vi "Main.vi"() -> ()   [LabVIEW 2020]
uses:
  <vilib>/Instr/_visa.llb/VISA Find Search Mode.ctl
  <vilib>/Platform/TimedLoop/XDataNode/timing_clust.ctl
  <vilib>/Platform/TimedLoop/XDataNode/nitl_modes.ctl
  <vilib>/Platform/TimedLoop/XDataNode/wakeup.ctl
  <vilib>/Platform/TimedLoop/scheduler/LVUserAPI/_suppVIs/Create_SoftwareTrigger_TSource.vi
  <vilib>/Platform/TimedLoop/scheduler/LVUserAPI/_suppVIs/Create_1kHz_TSource.vi
  <vilib>/platform/TimedLoop/XDataNode/XDataNode.xnode
  <vilib>/Platform/TimedLoop/XDataNode/XDNodeRunTimeDep.lvlib
panel:
  in  "Relay Mode":bool
  out "v1_1 13":bool=TRUE
  out "v1_1 12":bool=TRUE
  out "v1_1 11":bool=TRUE
  out "v1_1 10":bool=TRUE
  out "v1_1 9":bool=TRUE
  out "v1_1 8":bool=TRUE
  out "v1_1 7":bool=TRUE
  out "v1_1 6":bool=TRUE
  out "v1_1 5":bool=TRUE
  out "v1_1 4":bool=TRUE
  out "v1_1 3":bool=TRUE
  out "v1_1 2":bool=TRUE
  out "N2 4":bool caption="N2 2"
  out "N2 5":bool caption="N2 2"
  out "N2 3":bool caption="N2 2"
  out "Gas 11":bool
  out "Gas 10":bool
  out "Gas 9":bool
  out "H2O":bool
  out "CO2":bool
  out "CO":bool
  out "С2Н6":bool
  out "С2Н4":bool
  out "С2Н2":bool
  out "CH4":bool
  out "N2":bool
  out "v12_11":bool
  out "v12_10":bool
  out "v12_9":bool
  out "v12_8":bool
  out "v12_7":bool
  out "v12_6":bool
  out "v12_5":bool
  out "v12_4":bool
  out "v12_3":bool
  out "v12_2":bool
  out "v12_1":bool
  out "v4":bool
  out "flow 2":dbl format="%#.1f"
  out "v3_1":bool
  out "v3_2":bool
  out "v3_3":bool
  out "v2_3":bool
  out "v2_2":bool
  out "flow 1":dbl format="%#.1f"
  out "v2_1":bool
  out "v1_11":bool
  out "v1_10":bool
  out "v1_9":bool
  out "v1_8":bool
  out "v1_7":bool
  out "v1_6":bool
  out "v1_5":bool
  out "v1_4":bool
  out "v1_3":bool
  out "v1_2":bool
  out "v1_1":bool
  in  "coef":dbl(ring)=0.71 caption="Gas type" items=["NO2"=0.71, "SF6"=0.26]
  in  "Vlv_1 13":bool
  in  "Vlv_1 12":bool
  in  "Vlv_1 9":bool
  in  "Vlv_1 14":bool
  in  "DisableReadback":bool caption="Checkbox"
  out "Time left":i32
  in  "Stop":bool
  in  "Set point":i32
  in  "Play":bool
  in  "flow 2 s":dbl min=0.0 max=1000.0
  in  "flow 1 s":dbl min=0.0 max=500.0
  in  "Apply All":bool
  in  "Connect":bool
  in  "Vlv_1 11":bool
  in  "Vlv_1 8":bool
  in  "Vlv_1 7":bool
  in  "Vlv_1 6":bool
  in  "Vlv_1 5":bool
  in  "Vlv_1 4":bool
  in  "Vlv_1 3":bool
  in  "Vlv_1 2":bool
  in  "Vlv_1":bool
  in  "Vlv_1 10":bool
  out "Status":bool
  in  "CH2_SP":u16 max=999 step=1
  in  "CH1_SP":dbl max=999.0 step=1.0
  out "CH2_FB":u16=1 min=1 max=255 step=1
  out "CH1_FB":dbl=1.0 min=1.0 max=255.0 step=1.0 format="%.1g"
  out "Connection":bool
  out "find list":string[](array[string])
  in  "Port":u16(ring) items=["COM1 - Последовательный порт"]
  # "Current value"
  # "Gas 1 proportion"
  # "Gas 2 proportion"
  # "Current value"
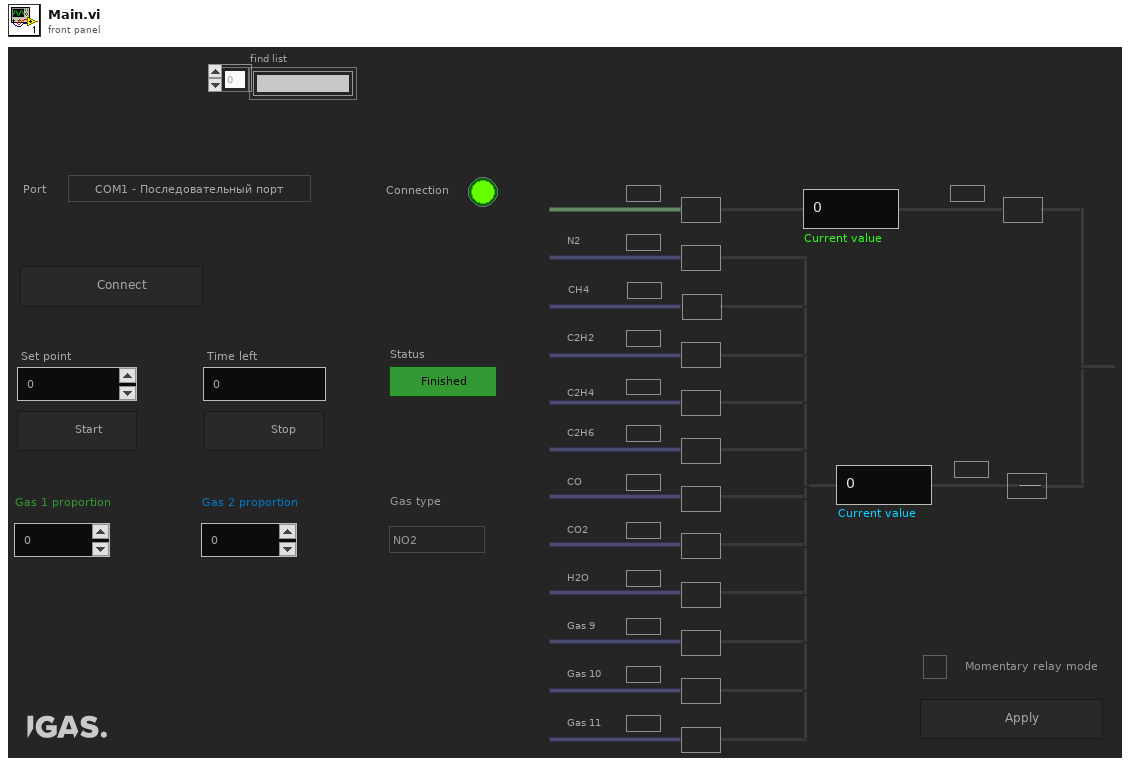
[diagram p1: front panel]
types:
  T1 = typedef "XDNodeRunTimeDep.lvlib/timing_clust.ctl" = cluster{"Expected End [f-1]":u64, "Actual End [f-1]":u64, "Finished Late? [f-1]":bool, "Expected End [i-1]":u64, "Actual End [i-1]":u64, "Finished Late? [i-1]":bool, "Expected Start [i]":u64, "Actual Start [i]":u64, "Expected Start [f]":u64, "Actual Start [f]":u64, "Source Name":string, "Structure Name":string, "Period":i64, "Deadline":i64, "Offset":i64, "Start":i64, "Priority":i32, "Timeout":i32, "Mode":T2, "Wakeup Reason":T3, "Error":errorcluster, "Source Type":string, "Secondary Source Type":string, "Global End Time":u64, "Global Start Time":u64, "Frame Duration":u64, "Iteration Duration":u64, "Assigned CPU":i32, "I/O Scan Engine Mode":u32}
  T2 = typedef "XDNodeRunTimeDep.lvlib/nitl_modes.ctl" = enum32{"No Change", "Process missed periods, maintain original phase", "Discard missed periods, maintain original phase", "Process missed periods, ignore original phase", "Discard missed periods, ignore original phase"}
  T3 = typedef "XDNodeRunTimeDep.lvlib/wakeup.ctl" = enum32{"Normal", "Aborted", "Asynchronous wakeup", "Timing source error", "Timed loop error", "Timeout"}
  T4 = cluster{"Mode":enum16{"RTU", "ASCII"}, "адрес датчика":u16}
  T5 = cluster{"Mode":enum16{"RTU", "ASCII"}, "Slave Address":u8}
  T6 = typedef "VISA Find Search Mode.ctl" = u32
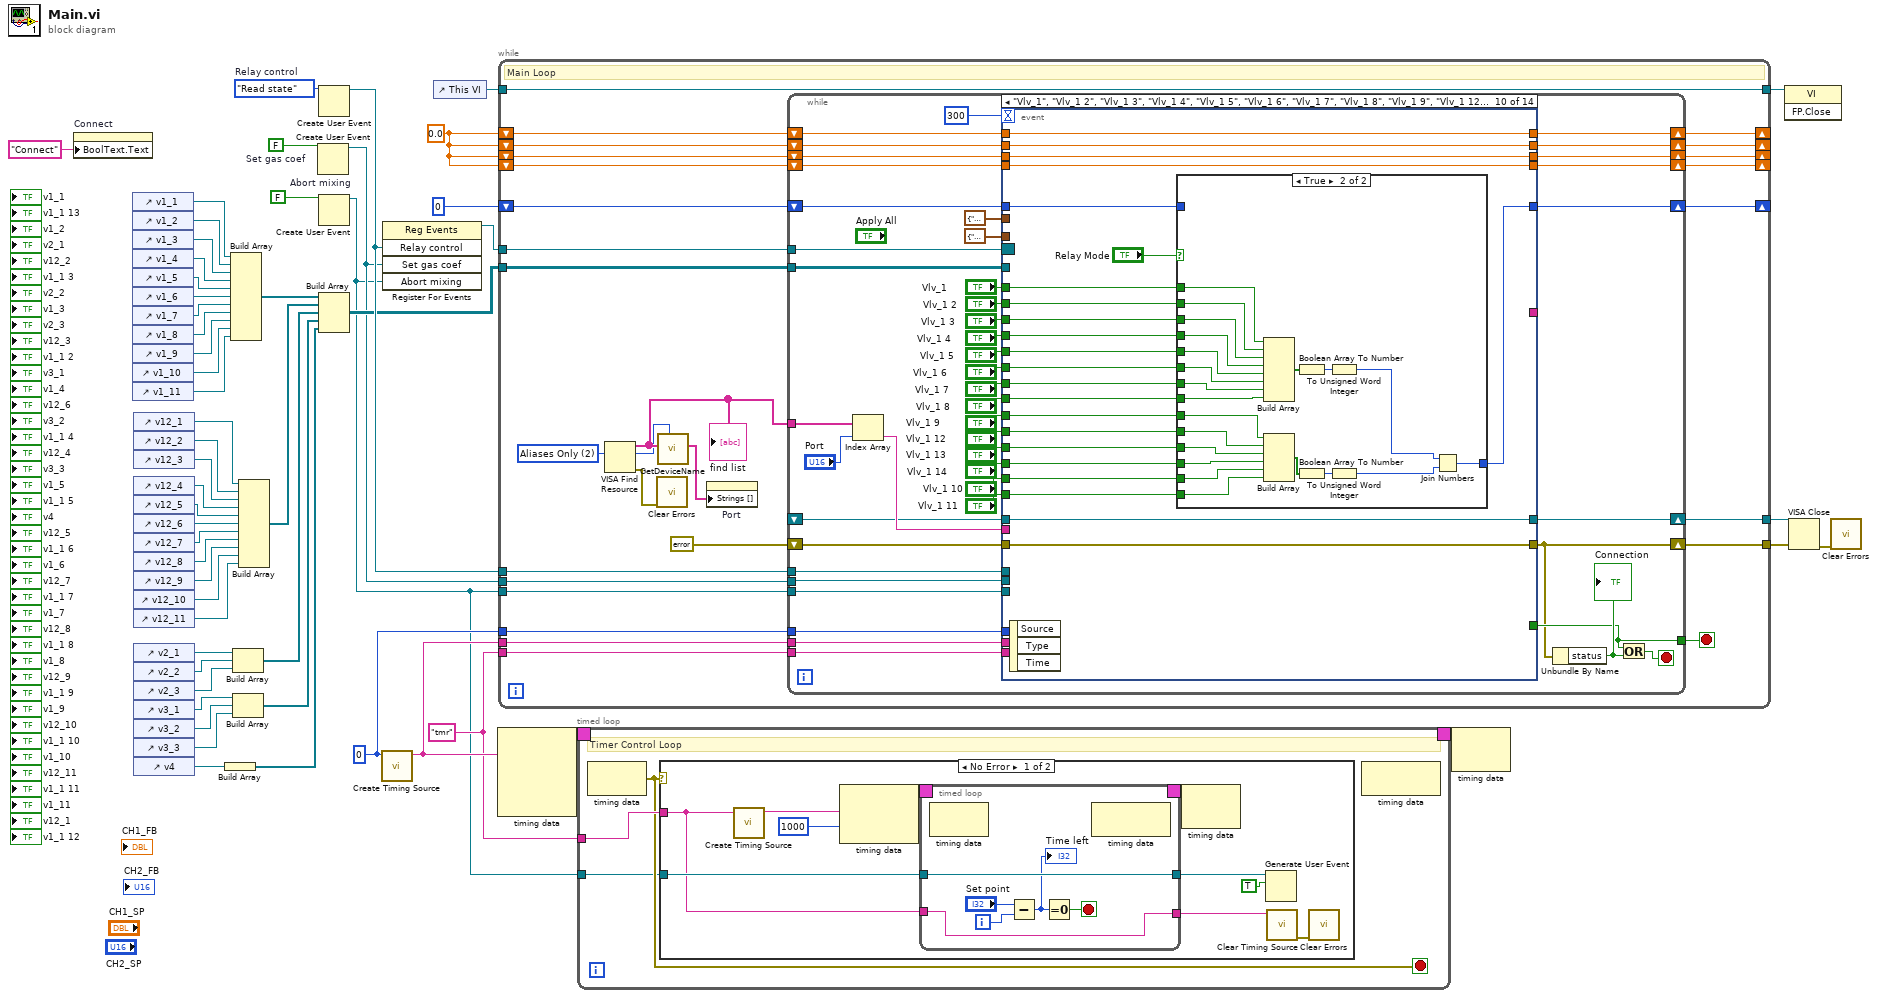
[diagram p0: block diagram]
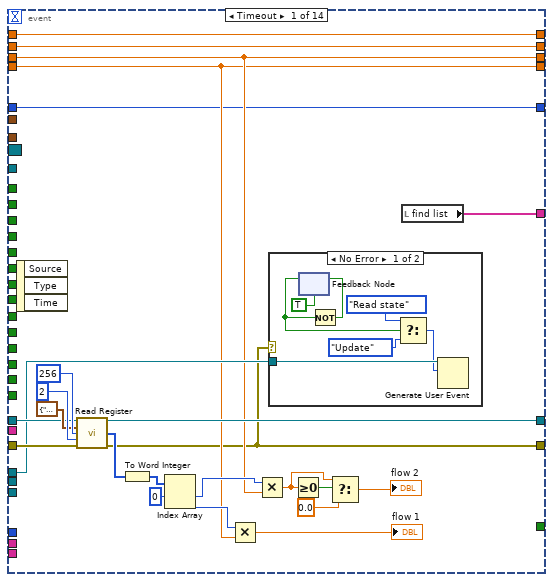
[diagram p3: hidden frame]
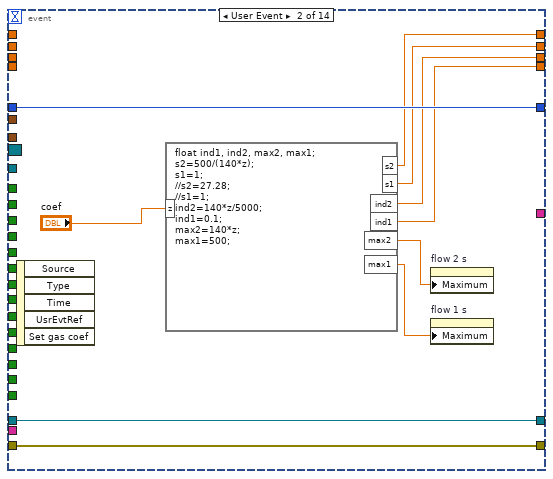
[diagram p5: hidden frame]
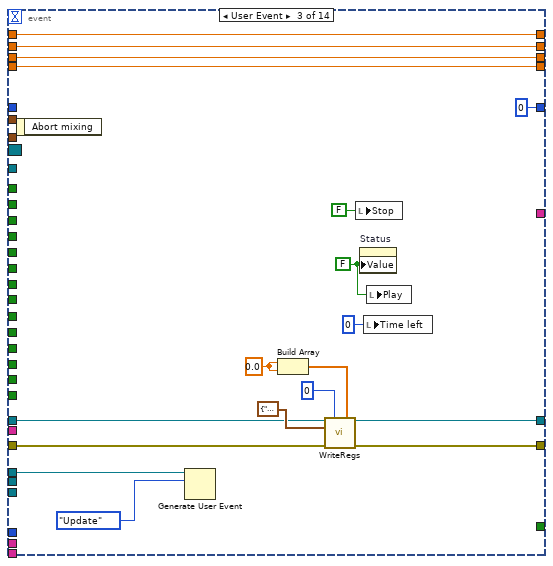
[diagram p6: hidden frame]
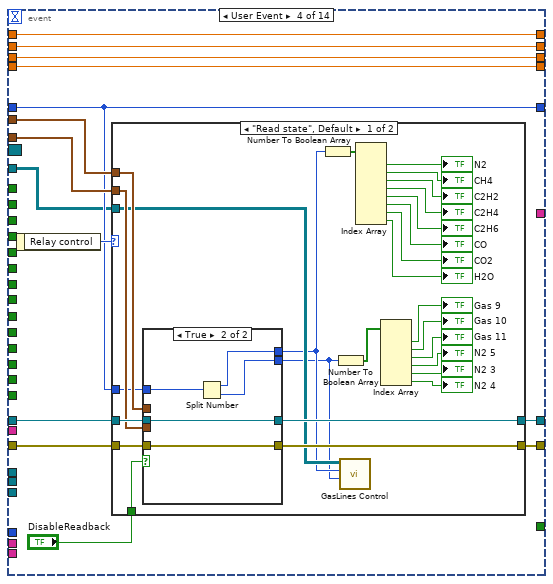
[diagram p7: hidden frame]
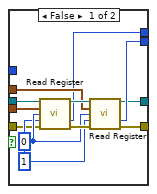
[diagram p8: hidden frame]
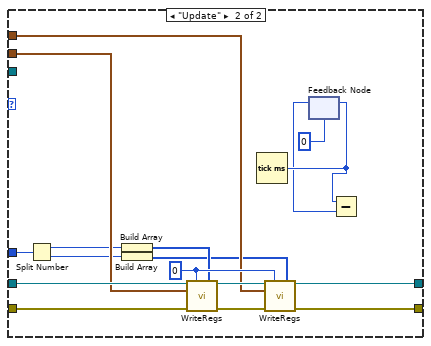
[diagram p9: hidden frame]
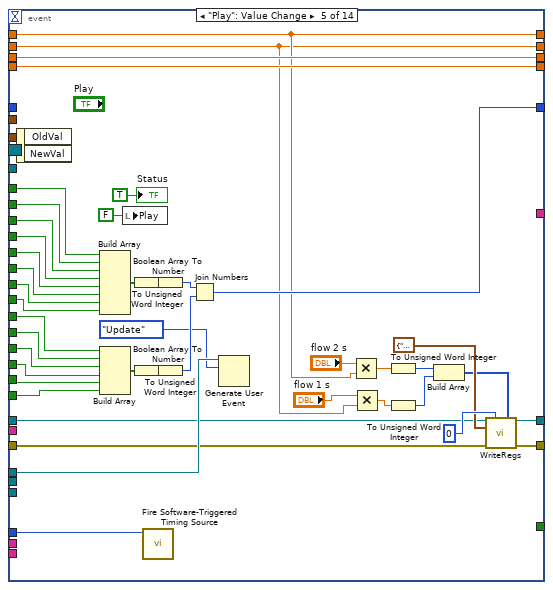
[diagram p10: hidden frame]
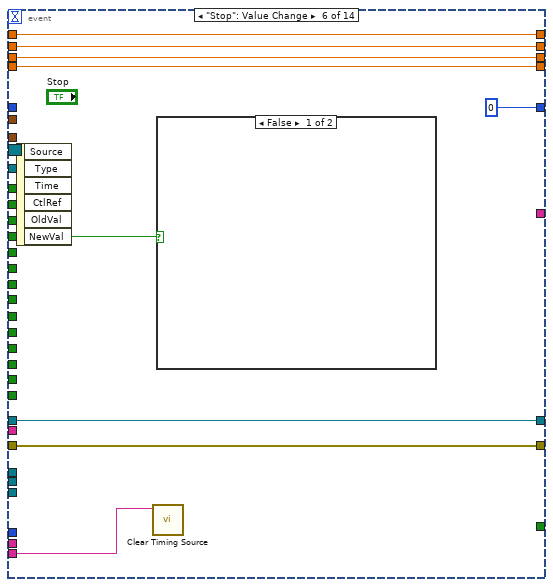
[diagram p11: hidden frame]
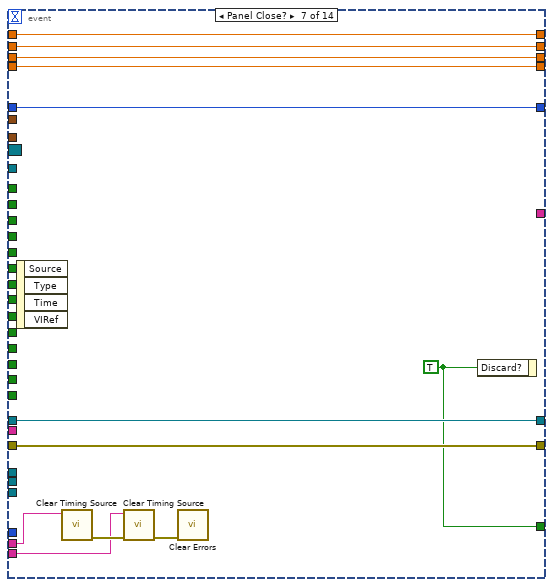
[diagram p13: hidden frame]
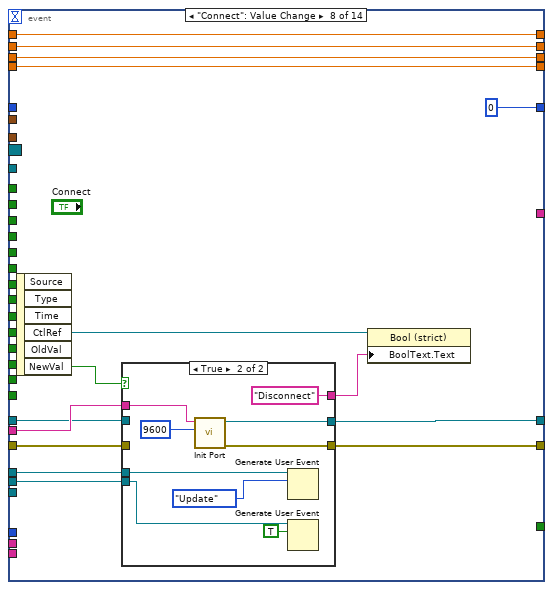
[diagram p14: hidden frame]
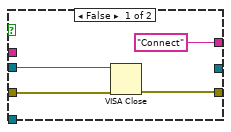
[diagram p15: hidden frame]
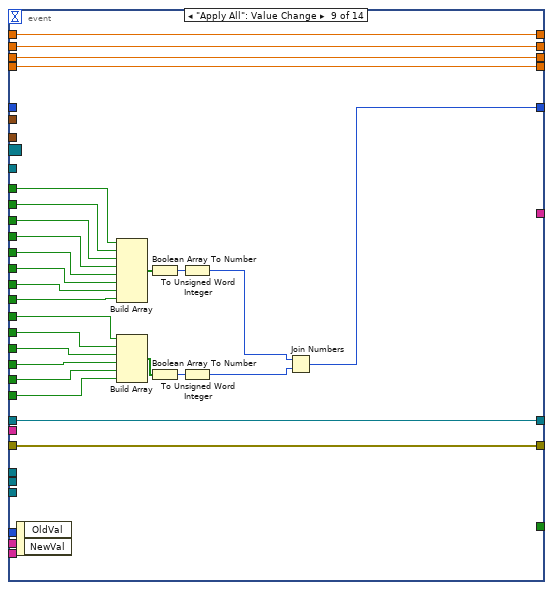
[diagram p16: hidden frame]
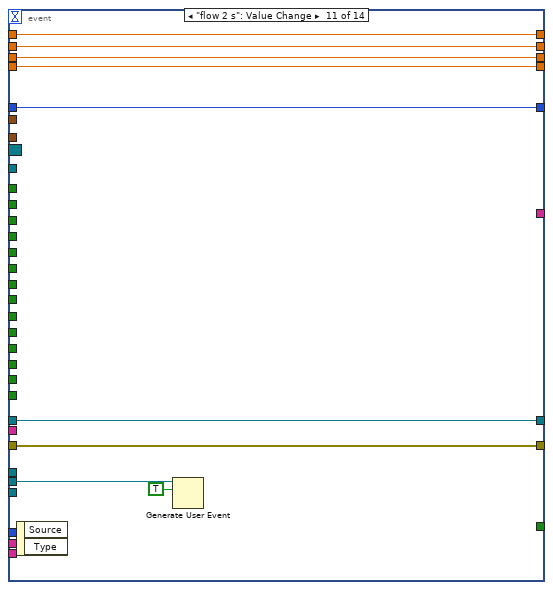
[diagram p18: hidden frame]
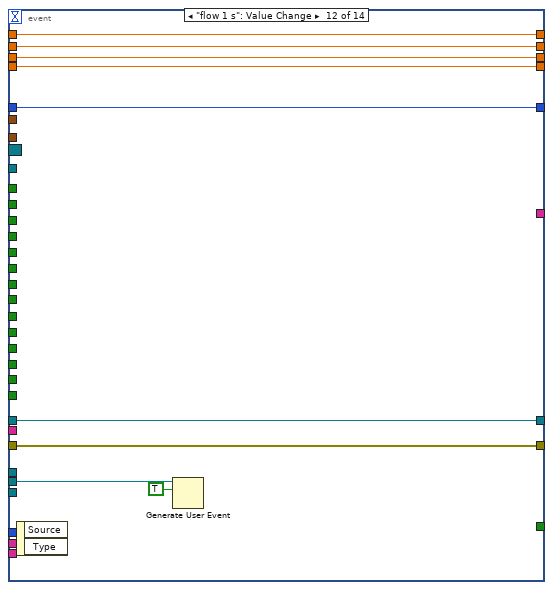
[diagram p19: hidden frame]
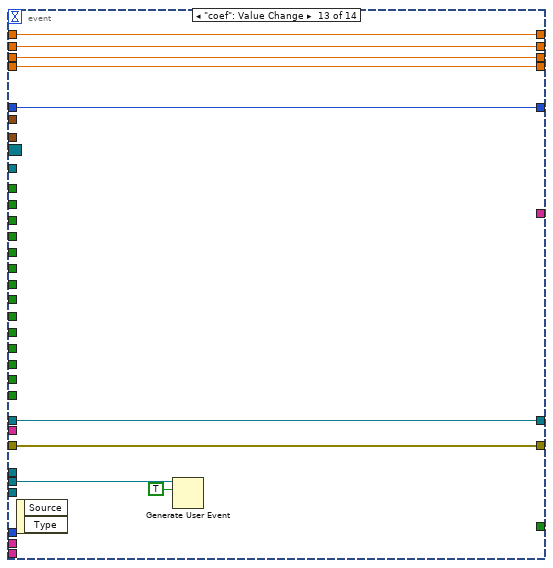
[diagram p20: hidden frame]
diagram:
  w3 = FALSE  # Abort mixing
  w4 = "tmr" ("name (in)")
  w6 = u8 0 ("trigger ID")
  w9 = 0.0 ("s2")
  w10 = FALSE  # Set gas coef
  w51 = enum16{"Read state", "Update"}."Read state"  # Relay control
  n1 = property on="Connect" class="Bool (strict)"("BoolText.Text"="Connect" ("Boolean Text.Text")) -> ()  [unwired: 2 in, 2 out]
  n2 = control-ref of="v1_1"() -> (w41:refnum<vi>)
  n3 = control-ref of="v1_2"() -> (w42:refnum<vi>)
  n4 = control-ref of="v1_3"() -> (w43:refnum<vi>)
  n5 = control-ref of="v1_4"() -> (w44:refnum<vi>)
  n6 = control-ref of="v1_5"() -> (w45:refnum<vi>)
  n7 = control-ref of="v1_6"() -> (w46:refnum<vi>)
  n8 = control-ref of="v1_7"() -> (w40:refnum<vi>)
  n9 = control-ref of="v1_8"() -> (w39:refnum<vi>)
  n10 = control-ref of="v1_9"() -> (w38:refnum<vi>)
  n11 = control-ref of="v1_10"() -> (w37:refnum<vi>)
  n12 = control-ref of="v1_11"() -> (w36:refnum<vi>)
  n13 = control-ref of="v12_1"() -> (w30:refnum<vi>)
  n14 = control-ref of="v12_2"() -> (w31:refnum<vi>)
  n15 = control-ref of="v12_3"() -> (w32:refnum<vi>)
  n16 = control-ref of="v12_4"() -> (w33:refnum<vi>)
  n17 = control-ref of="v12_5"() -> (w34:refnum<vi>)
  n18 = control-ref of="v12_6"() -> (w35:refnum<vi>)
  n19 = control-ref of="v12_7"() -> (w29:refnum<vi>)
  n20 = control-ref of="v12_8"() -> (w28:refnum<vi>)
  n21 = control-ref of="v12_9"() -> (w27:refnum<vi>)
  n22 = control-ref of="v12_10"() -> (w26:refnum<vi>)
  n23 = control-ref of="v12_11"() -> (w25:refnum<vi>)
  n24 = control-ref of="v2_1"() -> (w21:refnum<vi>)
  n25 = control-ref of="v2_2"() -> (w20:refnum<vi>)
  n26 = control-ref of="v2_3"() -> (w19:refnum<vi>)
  n27 = control-ref of="v3_1"() -> (w18:refnum<vi>)
  n28 = control-ref of="v3_2"() -> (w17:refnum<vi>)
  n29 = control-ref of="v3_3"() -> (w16:refnum<vi>)
  n30 = control-ref of="v4"() -> (w15:refnum<vi>)
  n31 = Build Array(w15) -> (w12:refnum<vi>[])
  n32 = Build Array(w41, w42, w43, w44, w45, w46, w40, w39, w38, w37, w36) -> (w24:refnum<vi>[])
  n33 = Build Array(w21, w20, w19) -> (w14:refnum<vi>[])
  n34 = Build Array(w18, w17, w16) -> (w13:refnum<vi>[])
  n35 = Build Array(w30, w31, w32, w33, w34, w35, w29, w28, w27, w26, w25) -> (w23:refnum<vi>[])
  n36 = Create User Event(user event datatype=w10) -> (user event=w2:refnum<user-event>)  [unwired: 1 in, 1 out]
  n37 = Create User Event(user event datatype=w51) -> (user event=w48:refnum<user-event>)  [unwired: 1 in, 1 out]
  n38 = Create User Event(user event datatype=w3) -> (user event=w1:refnum<user-event>)  [unwired: 1 in, 1 out]
  n39 = Build Array(w24, w23, w14, w13, w12) -> (w22:refnum<vi>[][])
  n40 = call-poly <vilib>:"Create Timing Source.vi"("trigger ID"=w6) -> ("timing source name"=w5:string)  [unwired: 9 in, 1 out]
  n41 = register-events(w48, w2, w1) -> (reference out=w50:refnum<event-registration>)  [unwired: 2 in, 1 out]
  n42 = control-ref of="This VI"() -> (w11:refnum<vi>)
  n43 = node-c288(w5) -> (w8:T1)  [unwired: 3 in]
  n44 = while {
    tunnel: [w69] -> w55
    tunnel: [w76] -> w54
    tunnel: [w75] -> w53
    tunnel: w50 -> [w74]
    shift-right: [w73] -> _
    shift-left: u32 0 -> [w72]
    tunnel: w48 -> [w71]
    tunnel: w22 -> [w70]
    tunnel: w11 -> [w69]
    shift-right: [w65] -> _
    shift-left: w9 -> [w67]
    shift-right: [w66] -> _
    shift-left: w9 -> [w68]
    shift-right: [w62] -> _
    shift-left: w9 -> [w64]
    shift-right: [w61] -> _
    shift-left: w9 -> [w63]
    tunnel: w2 -> [w60]
    tunnel: w6 -> [w59]
    tunnel: w5 -> [w58]
    tunnel: w4 -> [w56]
    tunnel: w1 -> [w57]
    stop <- w77 stop-if-true
    w80 = T6 2 items=["Canonical Names Only"=0, "Aliases Only"=2, "Include Matching Aliases"=3, "Include All Aliases"=4] ("Search Mode")
    # "Main Loop"
    n45 = VISA Find Resource(10:w80) -> (0:w78:errorcluster, 2:w81:u32, 3:w83:string[])  [unwired: 2 in]
    "find list" <- w83
    n46 = call <vilib>:"Clear Errors.vi"("error in (no error)"=w78) -> ()  [unwired: 5 in, 2 out]
    n47 = call "GetDeviceName.vi"("PortQuantity"=w81, "Input"=w83) -> ("Output"=w79:string[])  [unwired: 9 in]
    n48 = property on="Port" class="Ring (strict)"("Strings []"=w79) -> ()  [unwired: 2 in, 2 out]
    n49 = while {
      tunnel: w83 -> [w127]
      shift-right: [w98] -> w76
      shift-left: errorcluster {"status"=TRUE, "code"=0, "source"=""} ("error out") -> [w124]
      shift-right: [w122] -> w75
      shift-left: _ -> [w123]
      tunnel: [w107] -> w77
      tunnel: w74 -> [w106]
      shift-right: [w105] -> w73
      shift-left: w72 -> [w104]
      tunnel: w71 -> [w103]
      tunnel: w70 -> [w97]
      shift-right: [w96] -> w66
      shift-left: w68 -> [w89]
      shift-right: [w95] -> w65
      shift-left: w67 -> [w88]
      shift-right: [w92] -> w62
      shift-left: w64 -> [w94]
      shift-right: [w91] -> w61
      shift-left: w63 -> [w93]
      tunnel: w60 -> [w90]
      tunnel: w59 -> [w87]
      tunnel: w58 -> [w85]
      tunnel: w57 -> [w86]
      tunnel: w56 -> [w84]
      stop <- w109 stop-if-true
      n50 = Index Array(array=w127, index="Port") -> (element=w125:string)
      n51 = event shown="[9] \"Vlv_1\", \"Vlv_1 2\", \"Vlv_1 3\", \"Vlv_1 4\", \"Vlv_1 5\", \"Vlv_1 6\", \"Vlv_1 7\", \"Vlv_1 8\", \"Vlv_1 9\", \"Vlv_1 12\", \"Vlv_1 13\", \"Vlv_1 14\", \"Vlv_1 10\", \"Vlv_1 11\": Value Change" {
        selector: w106 -> [_ _ _ _ _ _ _ _ _ _ _ _ _ _]
        dyn-events: _ -> [_ _ _ _ _ _ _ _ _ _ _ _ _ _]
        timeout: 300 -> [_ _ _ _ _ _ _ _ _ _ _ _ _ _]
        tunnel: [w130 w169 w177 w197 w275 w312 w325 w340 w366 w393 w433 w442 w451 w459] -> w98
        tunnel: w125 -> [_ _ _ _ _ _ _ w341 _ _ _ _ _ _]
        tunnel: w124 -> [w146 w169 w178 w198 w273 w312 w325 w336 w366 w393 w433 w442 w451 w459]
        tunnel: [w138 w168 w176 w199 w276 w313 w326 w339 w367 w394 w434 w443 w452 w458] -> w122
        tunnel: w123 -> [w145 w168 w179 w200 w274 w313 w326 w337 w367 w394 w434 w443 w452 w458]
        tunnel: [w141 _ _ _ _ _ _ _ _ _ _ _ _ _] -> _
        tunnel: "Vlv_1" -> [_ _ _ _ w305 _ _ _ w381 w404 _ _ _ _]
        tunnel: "Vlv_1 2" -> [_ _ _ _ w304 _ _ _ w380 w403 _ _ _ _]
        tunnel: "Vlv_1 3" -> [_ _ _ _ w303 _ _ _ w379 w402 _ _ _ _]
        tunnel: "Vlv_1 4" -> [_ _ _ _ w302 _ _ _ w378 w401 _ _ _ _]
        tunnel: "Vlv_1 5" -> [_ _ _ _ w301 _ _ _ w377 w400 _ _ _ _]
        tunnel: "Vlv_1 6" -> [_ _ _ _ w300 _ _ _ w376 w399 _ _ _ _]
        tunnel: "Vlv_1 7" -> [_ _ _ _ w299 _ _ _ w375 w398 _ _ _ _]
        tunnel: "Vlv_1 8" -> [_ _ _ _ w298 _ _ _ w374 w397 _ _ _ _]
        tunnel: "Vlv_1 10" -> [_ _ _ _ w295 _ _ _ w371 w396 _ _ _ _]
        tunnel: "Vlv_1 11" -> [_ _ _ _ w294 _ _ _ w370 w395 _ _ _ _]
        tunnel: T4 {"Mode"=enum."RTU", "адрес датчика"=2} ("Mode") -> [_ _ _ w195 _ _ _ _ _ _ _ _ _ _]
        tunnel: T4 {"Mode"=enum."RTU", "адрес датчика"=1} ("Mode") -> [_ _ _ w196 _ _ _ _ _ _ _ _ _ _]
        tunnel: [_ _ _ _ _ _ w324 _ _ _ _ _ _ _] -> w107
        tunnel: [w129 w167 u32 0 ("t") w194 w297 u32 0 w323 u32 0 w363 w392 w435 w444 w453 w460] -> w105
        tunnel: w104 -> [w129 w167 _ w194 _ _ w323 _ _ w383 w435 w444 w453 w460]
        tunnel: w103 -> [w137 _ w171 _ w296 _ _ w332 _ _ _ _ _ _]
        tunnel: "Vlv_1 9" -> [_ _ _ _ w293 _ _ _ w359 w388 _ _ _ _]
        tunnel: "Vlv_1 12" -> [_ _ _ _ w292 _ _ _ w360 w389 _ _ _ _]
        tunnel: "Vlv_1 13" -> [_ _ _ _ w291 _ _ _ w361 w390 _ _ _ _]
        tunnel: "Vlv_1 14" -> [_ _ _ _ w290 _ _ _ w362 w391 _ _ _ _]
        tunnel: w97 -> [_ _ _ w192 _ _ _ _ _ _ _ _ _ _]
        tunnel: w89 -> [w134 _ w187 w191 w267 w310 w322 w331 w358 w387 w432 w441 w450 w457]
        tunnel: w88 -> [w133 _ w186 w190 w264 w309 w321 w330 w357 w386 w431 w440 w449 w456]
        tunnel: [w134 w166 w187 w191 w267 w310 w322 w331 w358 w387 w432 w441 w450 w457] -> w96
        tunnel: [w133 w165 w186 w190 w264 w309 w321 w330 w357 w386 w431 w440 w449 w456] -> w95
        tunnel: w94 -> [w132 _ w185 w189 w289 w308 w320 w329 w356 w385 w430 w439 w448 w455]
        tunnel: w93 -> [w131 _ w184 w188 w288 w307 w319 w328 w355 w384 w429 w438 w447 w454]
        tunnel: [w132 w164 w185 w189 w289 w308 w320 w329 w356 w385 w430 w439 w448 w455] -> w92
        tunnel: [w131 w163 w184 w188 w288 w307 w319 w328 w355 w384 w429 w438 w447 w454] -> w91
        tunnel: w90 -> [_ _ _ _ _ _ _ w327 _ _ w428 w437 w446 _]
        tunnel: w87 -> [_ _ _ _ w269 _ _ _ _ _ _ _ _ _]
        tunnel: w86 -> [_ _ _ _ _ _ _ _ _ _ _ _ _ _]
        tunnel: w85 -> [_ _ _ _ _ _ w318 _ _ _ _ _ _ _]
        tunnel: w84 -> [_ _ _ _ _ w306 w316 _ _ _ _ _ _ _]
        event Timeout {
          n52 = event-data() -> ()  [unwired: 1 in, 3 out]
          n53 = call "Read Register.vi"("Refnum in"=w145, "Mode"=T4 {"Mode"=enum."RTU", "адрес датчика"=3}, "startReg"=u16 256, "Quantity"=u16 2 ("startReg"), "error in (no error)"=w146) -> ("Refnum Out"=w138:refnum<visa-resource-name>, "Holding Registers"=w136:u16[], "error out"=w130:errorcluster)  [unwired: 6 in, 2 out]
          n54 = To Word Integer(number=w136) -> (16bit integer=w135:i16[])
          n55 = Index Array(array=w135, index #1=0 ("index")) -> (element #1=w151:i16, element #2=w152:i16)  [unwired: 1 in]
          n56 = Multiply(x=w152, y=w131) -> (x*y=→"flow 1":dbl)
          n57 = Multiply(x=w151, y=w132) -> (x*y=w143:dbl)
          n58 = case shown="No Error" w130 {
            tunnel: w137 -> [w159 _]
            frame No Error {
              n59 = feedback #1(TRUE) -> (w154:bool)
              n60 = Not(x=w154) -> (.not. x?=w153:bool)
              n61 = feedback-in #1(w153) -> ()
              n62 = Select(t=enum16{"Read state", "Update"}."Read state" ("event data"), s=w154, f=enum16{"Read state", "Update"}."Update" ("event data")) -> (s? t:f=w157:enum16{"Read state", "Update"})
              n63 = Generate User Event(user event=w159, event data cluster=w157) -> ()  [unwired: 2 in, 2 out]
            }
            frame Error {
            }
          }
          n64 = Greater Or Equal To 0?(x=w143) -> (x >= 0?=w144:bool)
          n65 = Select(t=w143, s=w144, f=0.0) -> (s? t:f=→"flow 2":dbl)
          n66 = local read "find list"() -> (w141:string[])
        }
        event User Event {
          n67 = event-data() -> ()  [unwired: 1 in, 5 out]
          n68 = formula code="float ind1, ind2, max2, max1;\ns2=500/(140*z);\ns1=1;\n//s2=27.28;\n//s1=1;\nind2=140*z/5000;\nind1=0.1;\nmax2=140*z;\nmax1=500;"("z"="coef") -> ("s2"=w166:dbl, "s1"=w165:dbl, "ind2"=w164:dbl, "ind1"=w163:dbl, "max2"=w161:dbl, "max1"=w160:dbl)
          n69 = property on="flow 2 s" class="DigNum (strict)"("Maximum"=w161) -> ()  [unwired: 2 in, 2 out]
          n70 = property on="flow 1 s" class="DigNum (strict)"("Maximum"=w160) -> ()  [unwired: 2 in, 2 out]
        }
        event User Event {
          w174 = FALSE ("Status")
          w182 = 0.0 ("x")
          n71 = event-data() -> ()  [unwired: 1 in, 1 out]
          n72 = Generate User Event(user event=w171, event data cluster=enum16{"Read state", "Update"}."Update" ("event data")) -> ()  [unwired: 2 in, 2 out]
          n73 = Build Array(w182, w182) -> (w183:dbl[])
          n74 = call "WriteRegs.vi"("VISA Refnum in"=w179, "StartAddr"=u16 0 ("Starting Address"), "DataArray"=w183, "Cluster"=T5 {"Mode"=enum."RTU", "Slave Address"=4} ("Serial Parameters"), "error in"=w178) -> ("VISA out"=w176:refnum<visa-resource-name>, "error out"=w177:errorcluster)  [unwired: 8 in, 1 out]
          n75 = local write "Stop"(FALSE ("Stop")) -> ()
          n76 = property on="Status" class="Bool (strict)"("Value"=w174) -> ()  [unwired: 2 in, 2 out]
          n77 = local write "Time left"(0 ("Time left")) -> ()
          n78 = local write "Play"(w174) -> ()
        }
        event User Event {
          n79 = event-data() -> ("Relay control"=w201:enum16{"Read state", "Update"})  [unwired: 1 in]
          n80 = case shown="\"Read state\", Default" w201 {
            tunnel: w200 -> [w220 w259]
            tunnel: [w219 w258] -> w199
            tunnel: w198 -> [w218 w257]
            tunnel: [w217 w256] -> w197
            tunnel: w196 -> [w216 w255]
            tunnel: w195 -> [w215 w254]
            tunnel: w194 -> [w213 w253]
            tunnel: "DisableReadback" -> [w214 _]
            tunnel: w192 -> [w204 _]
            frame "Read state", Default {
              n81 = case shown="True" w214 {
                tunnel: [w238 w241] -> w202
                tunnel: w220 -> [w235 w245]
                tunnel: [w234 w245] -> w219
                tunnel: w218 -> [w233 w244]
                tunnel: [w232 w244] -> w217
                tunnel: w216 -> [w231 _]
                tunnel: w215 -> [w230 _]
                tunnel: [w229 w242] -> w203
                tunnel: w213 -> [_ w243]
                frame False {
                  w236 = u16 1 ("Quantity")
                  w237 = u16 0 ("startReg")
                  n82 = call "Read Register.vi"("Refnum in"=w235, "Mode"=w231, "startReg"=w237, "Quantity"=w236, "error in (no error)"=w233) -> ("Refnum Out"=w240:refnum<visa-resource-name>, "Numeric"=w229:i16, "error out"=w239:errorcluster)  [unwired: 6 in, 2 out]
                  n83 = call "Read Register.vi"("Refnum in"=w240, "Mode"=w230, "startReg"=w237, "Quantity"=w236, "error in (no error)"=w239) -> ("Refnum Out"=w234:refnum<visa-resource-name>, "Numeric"=w238:i16, "error out"=w232:errorcluster)  [unwired: 6 in, 2 out]
                }
                frame True {
                  n84 = Split Number(x=w243) -> (hi(x)=w242:u16, lo(x)=w241:u16)
                }
              }
              n85 = Number To Boolean Array(number=w203) -> (Boolean array=w228:bool[])
              n86 = Number To Boolean Array(number=w202) -> (Boolean array=w224:bool[])
              n87 = call "GasLines Control.vi"("Numeric 2"=w202, "Numeric"=w203, "Array"=w204) -> ()  [unwired: 9 in]
              n88 = Index Array(array=w228) -> (element #1=→"N2":bool, element #2=→"CH4":bool, element #3=→"С2Н2":bool, element #4=→"С2Н4":bool, element #5=→"С2Н6":bool, element #6=→"CO":bool, element #7=→"CO2":bool, element #8=→"H2O":bool)  [unwired: 8 in]
              n89 = Index Array(array=w224) -> (element #1=→"Gas 9":bool, element #2=→"Gas 10":bool, element #3=→"Gas 11":bool, element #4=→"N2 5":bool, element #5=→"N2 3":bool, element #6=→"N2 4":bool)  [unwired: 6 in]
            }
            frame "Update" {
              w260 = u16 0 ("StartAddr")
              n90 = Split Number(x=w253) -> (hi(x)=w247:u16, lo(x)=w246:u16)
              n91 = Build Array(w247) -> (w252:u16[])
              n92 = Build Array(w246) -> (w251:u16[])
              n93 = call "WriteRegs.vi"("VISA Refnum in"=w259, "StartAddr"=w260, "DataArray"=w252, "Cluster"=w255, "error in"=w257) -> ("VISA out"=w262:refnum<visa-resource-name>, "error out"=w261:errorcluster)  [unwired: 8 in, 1 out]
              n94 = Tick Count (ms)() -> (millisecond timer value=w249:u32)
              n95 = call "WriteRegs.vi"("VISA Refnum in"=w262, "StartAddr"=w260, "DataArray"=w251, "Cluster"=w254, "error in"=w261) -> ("VISA out"=w258:refnum<visa-resource-name>, "error out"=w256:errorcluster)  [unwired: 8 in, 1 out]
              n96 = feedback-in #2(w249) -> ()
              n97 = feedback #2(u32 0 ("millisecond timer value")) -> (w248:u32)
              n98 = Subtract(x=w249, y=w248) -> ()  [unwired: 1 out]
            }
          }
        }
        event "Play": Value Change {
          n99 = event-data() -> ()  [unwired: 1 in, 2 out]
          n100 = Build Array(w305, w304, w303, w302, w301, w300, w299, w298) -> (w287:bool[])
          n101 = Build Array(w293, w292, w291, w290, w295, w294) -> (w284:bool[])
          n102 = local write "Play"(FALSE ("Play")) -> ()
          n103 = Boolean Array To Number(Boolean array=w287) -> (number=w286:u32)
          n104 = Boolean Array To Number(Boolean array=w284) -> (number=w285:u32)
          n105 = call <vilib>:"Fire Software-Triggered Timing Source.vi"("trigger ID"=w269) -> ()  [unwired: 9 in, 2 out]
          n106 = To Unsigned Word Integer(number=w286) -> (unsigned 16bit integer=w283:u16)
          n107 = To Unsigned Word Integer(number=w285) -> (unsigned 16bit integer=w282:u16)
          n108 = Join Numbers(hi=w283, lo=w282) -> ((hi.lo)=w297:u32)
          n109 = Generate User Event(user event=w296, event data cluster=enum16{"Read state", "Update"}."Update" ("event data")) -> ()  [unwired: 2 in, 2 out]
          n110 = Multiply(x="flow 2 s", y=w267) -> (x*y=w266:dbl)
          n111 = Multiply(x="flow 1 s", y=w264) -> (x*y=w265:dbl)
          n112 = To Unsigned Word Integer(number=w266) -> (unsigned 16bit integer=w279:u16)
          n113 = To Unsigned Word Integer(number=w265) -> (unsigned 16bit integer=w280:u16)
          n114 = Build Array(w279, w280) -> (w272:u16[])
          n115 = call "WriteRegs.vi"("VISA Refnum in"=w274, "StartAddr"=u16 0 ("Starting Address"), "DataArray"=w272, "Cluster"=T5 {"Mode"=enum."RTU", "Slave Address"=4} ("Serial Parameters"), "error in"=w273) -> ("VISA out"=w276:refnum<visa-resource-name>, "error out"=w275:errorcluster)  [unwired: 8 in, 1 out]
          "Status" <- TRUE ("Start")
        }
        event "Stop": Value Change {
          n116 = event-data() -> ("NewVal"=w311:bool)  [unwired: 1 in, 5 out]
          n117 = call <vilib>:"Clear Timing Source.vi"("name"=w306) -> ()  [unwired: 9 in, 2 out]
          n118 = case shown="False" w311 {
            frame False {
            }
            frame True {
            }
          }
        }
        event Panel Close? {
          w324 = TRUE ("Discard?")
          n119 = event-data() -> ()  [unwired: 1 in, 4 out]
          n120 = call <vilib>:"Clear Timing Source.vi"("name"=w318) -> ("error out"=w317:errorcluster)  [unwired: 9 in, 1 out]
          n121 = call <vilib>:"Clear Timing Source.vi"("error in (no error)"=w317, "name"=w316) -> ("error out"=w315:errorcluster)  [unwired: 8 in, 1 out]
          n122 = call <vilib>:"Clear Errors.vi"("error in (no error)"=w315) -> ()  [unwired: 5 in, 2 out]
          n123 = event-data("Discard?"=w324) -> ()  [unwired: 1 in, 1 out]
        }
        event "Connect": Value Change {
          n124 = event-data() -> ("CtlRef"=w335:refnum<vi>, "NewVal"=w338:bool)  [unwired: 1 in, 4 out]
          n125 = case shown="True" w338 {
            tunnel: w341 -> [_ w354]
            tunnel: [w343 w352] -> w340
            tunnel: [_ w351] -> w339
            tunnel: w337 -> [w345 _]
            tunnel: w336 -> [w344 _]
            tunnel: ["Connect" ("Boolean Text.Text") "Disconnect" ("Boolean Text.Text")] -> w334
            tunnel: w332 -> [_ w349]
            tunnel: w327 -> [_ w347]
            frame False {
              n126 = VISA Close(VISA resource name=w345, error in (no error)=w344) -> (error out=w343:errorcluster)
            }
            frame True {
              n127 = call "Init Port.vi"("BAUD"=u16 9600, "String"=w354) -> ("error out"=w352:errorcluster, "VISA Refnum out"=w351:refnum<visa-resource-name>)  [unwired: 8 in]
              n128 = Generate User Event(user event=w349, event data cluster=enum16{"Read state", "Update"}."Update" ("event data")) -> ()  [unwired: 2 in, 2 out]
              n129 = Generate User Event(user event=w347, event data cluster=TRUE ("event data")) -> ()  [unwired: 2 in, 2 out]
            }
          }
          n130 = property class="Bool (strict)"(reference=w335, "BoolText.Text"=w334) -> ()  [unwired: 1 in, 2 out]
        }
        event "Apply All": Value Change {
          n131 = event-data() -> ()  [unwired: 1 in, 2 out]
          n132 = Build Array(w381, w380, w379, w378, w377, w376, w375, w374) -> (w373:bool[])
          n133 = Build Array(w359, w360, w361, w362, w371, w370) -> (w368:bool[])
          n134 = Boolean Array To Number(Boolean array=w373) -> (number=w372:u32)
          n135 = Boolean Array To Number(Boolean array=w368) -> (number=w369:u32)
          n136 = To Unsigned Word Integer(number=w372) -> (unsigned 16bit integer=w365:u16)
          n137 = To Unsigned Word Integer(number=w369) -> (unsigned 16bit integer=w364:u16)
          n138 = Join Numbers(hi=w365, lo=w364) -> ((hi.lo)=w363:u32)
        }
        event "Vlv_1", "Vlv_1 2", "Vlv_1 3", "Vlv_1 4", "Vlv_1 5", "Vlv_1 6", "Vlv_1 7", "Vlv_1 8", "Vlv_1 9", "Vlv_1 12", "Vlv_1 13", "Vlv_1 14", "Vlv_1 10", "Vlv_1 11": Value Change {
          n139 = event-data() -> ()  [unwired: 1 in, 3 out]
          n140 = case shown="True" "Relay Mode" {
            tunnel: w404 -> [_ w426]
            tunnel: w403 -> [_ w425]
            tunnel: w402 -> [_ w424]
            tunnel: w401 -> [_ w423]
            tunnel: w400 -> [_ w422]
            tunnel: w399 -> [_ w421]
            tunnel: w398 -> [_ w420]
            tunnel: w397 -> [_ w419]
            tunnel: w396 -> [_ w416]
            tunnel: w395 -> [_ w415]
            tunnel: [w405 w410] -> w392
            tunnel: w391 -> [_ w409]
            tunnel: w390 -> [_ w408]
            tunnel: w389 -> [_ w407]
            tunnel: w388 -> [_ w406]
            tunnel: w383 -> [w405 _]
            frame False {
            }
            frame True {
              n141 = Build Array(w426, w425, w424, w423, w422, w421, w420, w419) -> (w418:bool[])
              n142 = Build Array(w406, w407, w408, w409, w416, w415) -> (w413:bool[])
              n143 = Boolean Array To Number(Boolean array=w418) -> (number=w417:u32)
              n144 = Boolean Array To Number(Boolean array=w413) -> (number=w414:u32)
              n145 = To Unsigned Word Integer(number=w417) -> (unsigned 16bit integer=w412:u16)
              n146 = To Unsigned Word Integer(number=w414) -> (unsigned 16bit integer=w411:u16)
              n147 = Join Numbers(hi=w412, lo=w411) -> ((hi.lo)=w410:u32)
            }
          }
        }
        event "flow 2 s": Value Change {
          n148 = event-data() -> ()  [unwired: 1 in, 2 out]
          n149 = Generate User Event(user event=w428, event data cluster=TRUE ("event data")) -> ()  [unwired: 2 in, 2 out]
        }
        event "flow 1 s": Value Change {
          n150 = event-data() -> ()  [unwired: 1 in, 2 out]
          n151 = Generate User Event(user event=w437, event data cluster=TRUE ("event data")) -> ()  [unwired: 2 in, 2 out]
        }
        event "coef": Value Change {
          n152 = event-data() -> ()  [unwired: 1 in, 2 out]
          n153 = Generate User Event(user event=w446, event data cluster=TRUE ("event data")) -> ()  [unwired: 2 in, 2 out]
        }
        event "Port": Mouse Down {
          n154 = event-data() -> ()  [unwired: 1 in, 8 out]
        }
      }
      n155 = Unbundle By Name(w98) -> ("status"=w108:bool)
      "Connection" <- w108
      n156 = Or(x=w107, y=w108) -> (x .or. y?=w109:bool)
    }
  }
  n157 = timed-loop {
    timing: w8 -> [_]
    timing-out: [_] -> w7
    tunnel: w4 -> [w463]
    tunnel: w1 -> [w461]
    stop <- w462 stop-if-true
    # "Timer Control Loop"
    n158 = node-c288() -> (w462:errorcluster)  [unwired: 1 in]
    n159 = case shown="No Error" w462 {
      tunnel: w463 -> [w466 _]
      tunnel: w461 -> [w469 _]
      frame No Error {
        n160 = call-poly <vilib>:"Create Timing Source.vi"("name (in)"=w466) -> ("name (out)"=w470:string)  [unwired: 9 in, 1 out]
        n161 = node-c288(w470, i64 1000 ("Period")) -> (w473:T1)
        n162 = timed-loop {
          timing: w473 -> [_]
          timing-out: [_] -> w472
          tunnel: [w477] -> w467
          tunnel: w469 -> [w477]
          tunnel: w466 -> [w474]
          tunnel: [w474] -> w465
          i -> [w479]
          stop <- w478 stop-if-true
          n163 = node-c288() -> ()  [unwired: 1 in, 1 out]
          n164 = Subtract(x="Set point", y=w479) -> (x-y=w475:i32)
          "Time left" <- w475
          n165 = Equal To 0?(x=w475) -> (x = 0?=w478:bool)
          n166 = node-c288() -> ()  [unwired: 1 in, 1 out]
        }
        n167 = node-c288(w472) -> ()  [unwired: 1 out]
        n168 = Generate User Event(user event=w467, event data cluster=TRUE ("event data")) -> ()  [unwired: 2 in, 2 out]
        n169 = call <vilib>:"Clear Timing Source.vi"("name"=w465) -> ("error out"=w464:errorcluster)  [unwired: 9 in, 1 out]
        n170 = call <vilib>:"Clear Errors.vi"("error in (no error)"=w464) -> ()  [unwired: 5 in, 2 out]
      }
      frame Error {
      }
    }
    n171 = node-c288() -> ()  [unwired: 1 in, 1 out]
  }
  n172 = node-c288(w7) -> ()  [unwired: 1 out]
  n173 = invoke class="VI" method="FP.Close"(reference=w55) -> ()  [unwired: 2 in, 3 out]
  n174 = VISA Close(VISA resource name=w53, error in (no error)=w54) -> (error out=w52:errorcluster)
  n175 = call <vilib>:"Clear Errors.vi"("error in (no error)"=w52) -> ()  [unwired: 5 in, 2 out]
